vi "Test of the EMP PM.vi"() -> ()   [LabVIEW 2020, in "PM-EMP.lvclass"]
uses:
  PM-EMP.lvclass
  C:/Sandbox/Git_Sandbox/WiSpry Test Framework source code (LV20)/WiSpry Test Framework/Instruments/Instrument.lvclass
  Instrument.lvclass/Instrument.ctl
  Instrument.lvclass
panel:
  out "Power Out":dbl[](array[numeric])
  out "error out":errorcluster
  in  "VISA resource name":refnum<visa-resource-name>
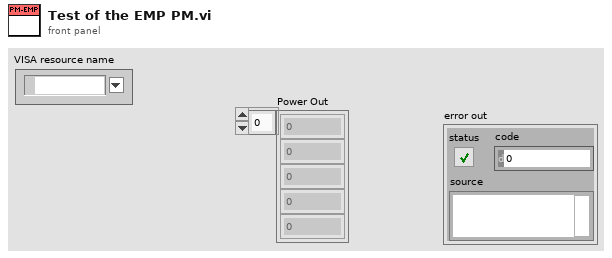
[diagram p1: front panel]
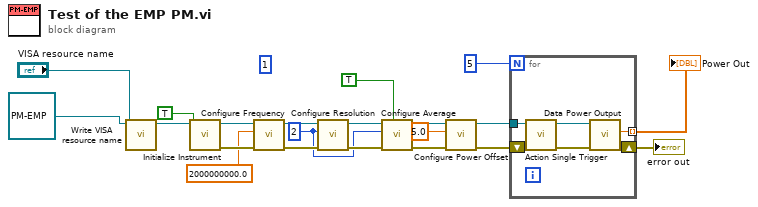
[diagram p0: block diagram]
diagram:
  (unwired) u16 1 ("Channel")
  w9 = 2 ("Resolution")
  n1 = call "Write VISA resource name.vi"("VISA resource name"="VISA resource name", "Instrument in"=refnum<class "PM-EMP.lvclass"> refnum ("PM-EMP.lvclass")) -> ("Instrument out"=w19:refnum<class "PM-EMP.lvclass">)  [unwired: 9 in]
  n2 = call-dynamic "Initialize Instrument.vi"("Reset"=TRUE, "PM-EMP in"=w19) -> ("error out"=w17:errorcluster, "PM-EMP out"=w16:refnum<class "PM-EMP.lvclass">)  [unwired: 8 in]
  n3 = call-dynamic "Configure Frequency.vi"("error in (no error)"=w17, "Frequency"=2000000000.0, "PM-EMP in"=w16) -> ("error out"=w13:errorcluster, "PM-EMP out"=w14:refnum<class "PM-EMP.lvclass">)  [unwired: 7 in]
  n4 = call-dynamic "Configure Resolution.vi"("error in (no error)"=w13, "Resolution"=w9, "PM-EMP in"=w14) -> ("error out"=w12:errorcluster, "PM-EMP out"=w11:refnum<class "PM-EMP.lvclass">)  [unwired: 7 in]
  n5 = call-dynamic "Configure Average.vi"("Average on"=TRUE, "error in (no error)"=w12, "Average Count"=w9, "PM-EMP in"=w11) -> ("error out"=w6:errorcluster, "PM-EMP out"=w5:refnum<class "PM-EMP.lvclass">)  [unwired: 6 in]
  n6 = call-dynamic "Configure Power Offset.vi"("error in (no error)"=w6, "Power Offset"=5.0, "PM-EMP in"=w5) -> ("error out"=w3:errorcluster, "PM-EMP out"=w2:refnum<class "PM-EMP.lvclass">)  [unwired: 7 in]
  n7 = for {
    N: 5 -> [_]
    tunnel: w2 -> [w26]
    tunnel: [w23] -> w1 mode=indexing
    shift-right: [w22] -> w7
    shift-left: w3 -> [w27]
    n8 = call-dynamic "Action Single Trigger.vi"("error in (no error)"=w27, "PM-EMP in"=w26) -> ("error out"=w25:errorcluster, "PM-EMP out"=w24:refnum<class "PM-EMP.lvclass">)  [unwired: 8 in]
    n9 = call-dynamic "Data Power Output.vi"("error in (no error)"=w25, "PM-EMP in"=w24) -> ("error out"=w22:errorcluster, "Power Out"=w23:dbl)  [unwired: 7 in, 1 out]
  }
  "error out" <- w7
  "Power Out" <- w1
